vi "Insert_NewHeaders.vi"(8 "error in":errorcluster, 9 "Array In":string[](array[string]), 10 "Headers":string[](array[string])=["Numeric Data", "Float Data", "String Data", "Enum Data", "Array Data[0].Numeric Data", "Array Data 2[0].Numeric Data", "Array Data 2[1].Numeric Data"], 11 "refnum out":refnum<file>) -> (0 "error out":errorcluster, 2 "Result":bool)   [LabVIEW 2014, in "TableLogger_CSV_Actor.lvlib" / "TableLogger_CSV_Actor.lvclass"]
uses:
  TableLogger_CSV_Actor.lvclass
panel:
  # "Connector Pane"
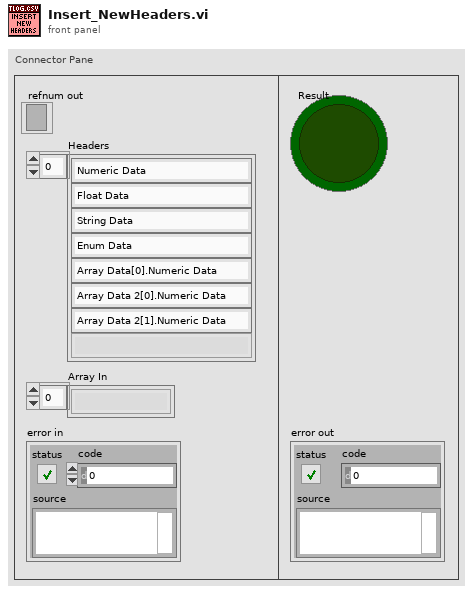
[diagram p1: front panel]
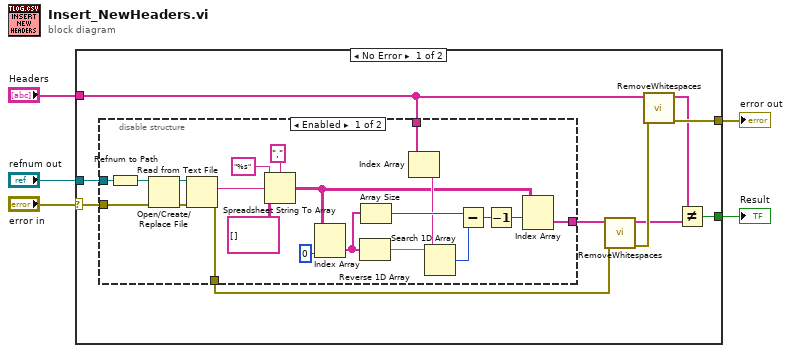
[diagram p0: block diagram]
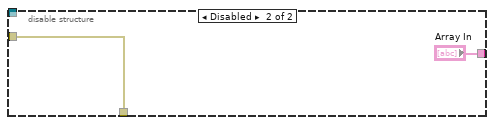
[diagram p2: hidden frame]
diagram:
  n1 = case shown="No Error" "error in" {
    selector: "error in" -> [w7 w38]
    tunnel: "Headers" -> [w14 _]
    tunnel: [w11 w38] -> w4
    tunnel: [w10 _] -> w3
    tunnel: "refnum out" -> [w6 _]
    frame No Error {
      n2 = disable-structure shown="Enabled" {
        disable-tunnel: [w26 "Array In"] -> w15
        disable-tunnel: w14 -> [w25 _]
        disable-tunnel: [w23 w36] -> w13
        disable-tunnel: w7 -> [w20 w36]
        disable-tunnel: w6 -> [w16 _]
        frame Enabled {
          n3 = Refnum to Path(1:w16) -> (0:w17:path)
          n4 = Open/Create/Replace File(file path (use dialog)=w17) -> (refnum out=w18:refnum<file>)  [unwired: 5 in, 2 out]
          n5 = Read from Text File(file (use dialog)=w18, error in=w20) -> (text=w19:string, error out=w23:errorcluster)  [unwired: 2 in, 2 out]
          n6 = Spreadsheet String To Array(delimiter (Tab)=",", format string="%s", spreadsheet string=w19, array type (2D Dbl)=string[][] []) -> (array=w24:string[][])
          n7 = Index Array(array=w24, index (col)=0 ("disabled index (col)")) -> (element=w30:string[])  [unwired: 1 in]
          n8 = Reverse 1D Array(array=w30) -> (reversed array=w31:string[])
          n9 = Array Size(array=w30) -> (size(s)=w29:i32)
          n10 = Index Array(array=w25) -> (element=w28:string)  [unwired: 1 in]
          n11 = Search 1D Array(1D array=w31, element=w28) -> (index of element=w27:i32)  [unwired: 1 in]
          n12 = Subtract(x=w29, y=w27) -> (x-y=w22:i32)
          n13 = Decrement(x=w22) -> (x-1=w21:i32)
          n14 = Index Array(array=w24, index (row)=w21) -> (element=w26:string[])  [unwired: 1 in]
        }
        frame Disabled {
        }
      }
      n15 = call "RemoveWhitespaces.vi"("error in (no error)"=w13, "Array In"=w15) -> ("error out"=w12:errorcluster, "Array removing empty space"=w8:string[])  [unwired: 8 in]
      n16 = call "RemoveWhitespaces.vi"("error in (no error)"=w12, "Array In"=w14) -> ("error out"=w11:errorcluster, "Array removing empty space"=w9:string[])  [unwired: 8 in]
      n17 = Not Equal?(x=w9, y=w8) -> (x != y?=w10:bool)
    }
    frame Error {
    }
  }
  "error out" <- w4
  "Result" <- w3
